vi "runtest increment seqcount.vi"(3 "POST (empty)":T1) -> (1 "new POST":T1)   [LabVIEW 2011]
uses:
  ITK EXT/utils/keyedarr.llb/Keyed Array.ctl
  ITK EXT/utils/strutil.llb/Case Matching.ctl
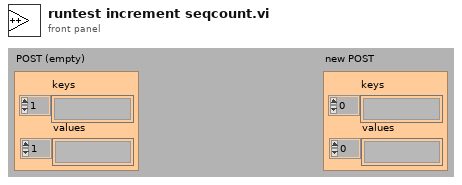
[diagram p1: front panel]
types:
  T1 = typedef "Keyed Array.ctl" = cluster{"keys":string[], "values":string[]}
  T2 = typedef "Case Matching.ctl" = enum16{"a != A", "a == A", "system"}
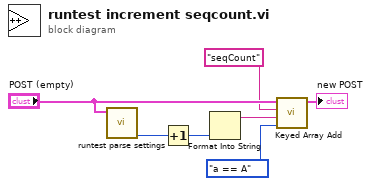
[diagram p0: block diagram]
diagram:
  n1 = call "runtest parse settings.vi"("POST (empty)"="POST (empty)") -> ("SeqCount"=w4:i32)  [unwired: 10 out]
  n2 = Increment(x=w4) -> (x+1=w2:i32)
  n3 = Format Into String(w2) -> (resulting string=w1:string)  [unwired: 3 in, 1 out]
  n4 = call "Keyed Array Add.vi"("case matching (sensitive)"=Case_Matching."a == A", "value"=w1, "key"="seqCount", "array in"="POST (empty)") -> ("array out"=→"new POST":T1)  [unwired: 3 out]
